vi "N4_X01_Query.vi"(5 "Delay Befor (s)":T7=0.5, 7 "Command":T8, 8 "error in":T9, 11 "DriverConnect in":T1={"InterfaceType"=enum."VISA", "OpenedSession"="", "InterfaceSettings"={"Interface"=enum."RS232", "EOS 4 read"=enum."LF (\\n)", "EOS 4 write"=enum."LF (\\n)", "TMO, ms"=10000, "Sett"=variant(cluster{"Baud Rate":u32, "Data Bits":u16, "Parity":u16, "Stop Bits":u16, "Flow Control":u16, "Eho":bool} {"Baud Rate"=75, "Data Bits"=0, "Parity"=0, "Stop Bits"=0, "Flow Control"=0, "Eho"=FALSE})}}) -> (0 "error out":T9, 3 "DriverConnect out":T1={"InterfaceType"=enum."VISA", "OpenedSession"="", "InterfaceSettings"={"Interface"=enum."RS232", "EOS 4 read"=enum."LF (\\n)", "EOS 4 write"=enum."LF (\\n)", "TMO, ms"=10000, "Sett"=variant(cluster{"Baud Rate":u32, "Data Bits":u16, "Parity":u16, "Stop Bits":u16, "Flow Control":u16, "Eho":bool} {"Baud Rate"=75, "Data Bits"=0, "Parity"=0, "Stop Bits"=0, "Flow Control"=0, "Eho"=FALSE})}}, 6 "Response":T6)   [LabVIEW 2018]
uses:
  MOKO_LabViewLibrary/MokoLowLevel/MokoLowLovelControl/MLLC_Error.ctl
  MOKO_LabViewLibrary/MokoLowLevel/MokoLowLovelControl/MLLC_Command.ctl
  MOKO_LabViewLibrary/MokoLowLevel/MokoLowLovelControl/MLLC_Delay.ctl
  MOKO_LabViewLibrary/MokoLowLevel/MokoLowLovelControl/MLLC_Response.ctl
  MOKO_LabViewLibrary/MokoLowLevel/MokoLowLovelControl/MLLC_ConnectCluster.ctl
  MOKO_LabViewLibrary/MokoLowLevel/MokoLowLovelControl/MLLC_InterfaceType.ctl
  MOKO_LabViewLibrary/MokoLowLevel/MokoLowLovelControl/MLLC_OpenedSession.ctl
  MOKO_LabViewLibrary/MokoLowLevel/MokoLowLovelControl/MLLC_InterfaceSettings.ctl
  MOKO_LabViewLibrary/MokoLowLevel/MokoLowLovelControl/MLLC_InterfaceKind.ctl
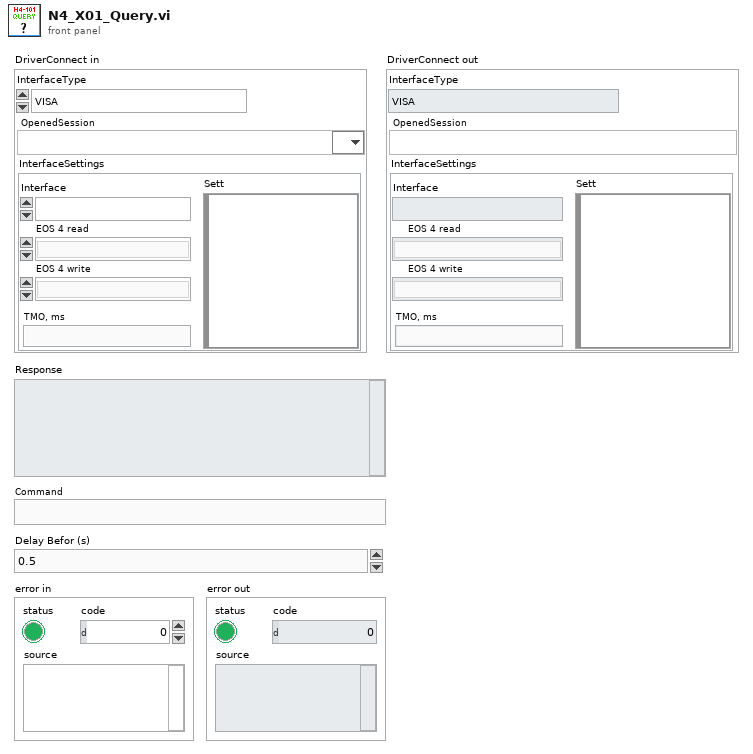
[diagram p1: front panel]
types:
  T1 = typedef "MLLC_ConnectCluster.ctl" = cluster{"InterfaceType":T2, "OpenedSession":T3, "InterfaceSettings":T4}
  T2 = typedef "MLLC_InterfaceType.ctl" = enum16{"VISA", "Prologix USB-GPIB"}
  T3 = typedef "MLLC_OpenedSession.ctl" = refnum<visa-resource-name>
  T4 = typedef "MLLC_InterfaceSettings.ctl" = cluster{"Interface":T5, "EOS 4 read":enum16{"Default (=EOS 4 write)", "CR (\\r)", "LF (\\n)", "None"}, "EOS 4 write":enum16{"CR+LF (\\r\\n)", "CR (\\r)", "LF (\\n)", "None"}, "TMO, ms":i32, "Sett":variant}
  T5 = typedef "MLLC_InterfaceKind.ctl" = enum16{"RS232", "GPIB", "USB", "Ethernet", "another"}
  T6 = typedef "MLLC_Response.ctl" = string
  T7 = typedef "MLLC_Delay.ctl" = dbl
  T8 = typedef "MLLC_Command.ctl" = string
  T9 = typedef "MLLC_Error.ctl" = errorcluster
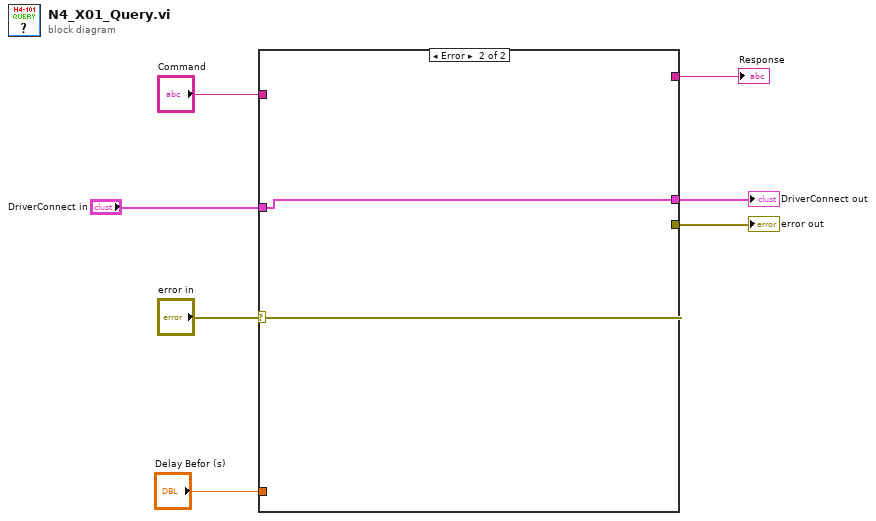
[diagram p0: block diagram]
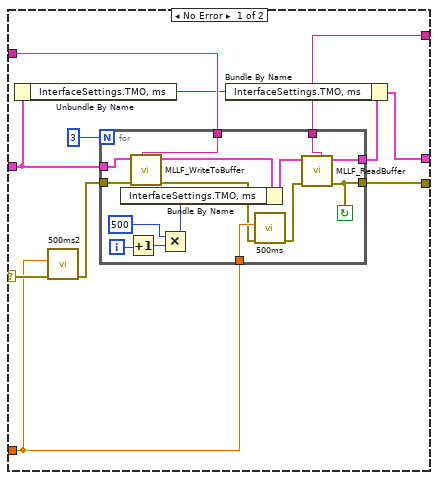
[diagram p2: hidden frame]
diagram:
  n1 = case shown="Error" "error in" {
    selector: "error in" -> [w17 w35]
    tunnel: [w15 w35] -> w7
    tunnel: [w8 w34] -> w1
    tunnel: "DriverConnect in" -> [w11 w34]
    tunnel: "Command" -> [w18 _]
    tunnel: "Delay Befor (s)" -> [w10 _]
    tunnel: [w13 _] -> w3
    frame No Error {
      n2 = Unbundle By Name(w11) -> ("InterfaceSettings.TMO, ms"=w14:i32)
      n3 = call "500ms2"("error in (no error)"=w17, "Delay Time (s)"=w10) -> ("error out"=w16:errorcluster)  [unwired: 9 in]
      n4 = for {
        N: 3 -> [_]
        tunnel: w18 -> [w33]
        tunnel: w16 -> [w32]
        tunnel: [w31] -> w9
        tunnel: [w25] -> w15
        tunnel: w11 -> [w21]
        tunnel: [w30] -> w13
        tunnel: w10 -> [w24]
        i -> [w29]
        stop <- w25 continue-if-true
        n5 = Increment(x=w29) -> (x+1=w28:i32)
        n6 = call "MLLF_WriteToBuffer.vi"("String"=w33, "error in"=w32, "DriverConnect in"=w21) -> ("error out"=w22:T9, "DriverConnect out"=w20:T1)  [unwired: 5 in]
        n7 = Multiply(x=500 ("TMO, ms"), y=w28) -> (x*y=w26:i32)
        n8 = Bundle By Name(cluster=w20, "InterfaceSettings.TMO, ms"=w26) -> (w19:T1)
        n9 = call "500ms"("error in (no error)"=w22, "Delay Time (s)"=w24) -> ("error out"=w23:errorcluster)  [unwired: 9 in]
        n10 = call "MLLF_ReadBuffer.vi"("Error In"=w23, "DriverConnect in"=w19) -> ("Error Out"=w25:errorcluster, "DriverConnect out"=w31:T1, "String"=w30:string)  [unwired: 6 in]
      }
      n11 = Bundle By Name(cluster=w9, "InterfaceSettings.TMO, ms"=w14) -> (w8:T1)
    }
    frame Error {
    }
  }
  "error out" <- w7
  "Response" <- w3
  "DriverConnect out" <- w1
